vi "Load Reference.vi"(8 "error in (no error)":errorcluster, 10 "Reference":refnum<vi>, 11 "LargeScrollbar in":refnum<class "LargeScrollbar.lvclass">) -> (0 "error out":errorcluster, 3 "LargeScrollbar out":refnum<class "LargeScrollbar.lvclass">)   [LabVIEW 2015, in "LargeScrollbar.lvclass"]
doc: "The <b>Load Reference VI</b> is a dynamic dispatch VI that must be overwritten in every QControl Class and must <b>Call Parent Method</b>. This recursively loads the reference of the control to the data space for the Control Class up the inheritance hierarchy (class hierarchy). These references must be loaded in this way to use all of the built-in properties.\n\nThe reference input is the reference type needed for the control but is coerced to Generic. It should be cast back to the correct type before bundling into the class private data. The pre-casted \"Generic\" reference is wired as input to the <b>Call Parent Method</b>.\n<b> </b> <b> </b>\n©2016 Q Software Innovations, LLC (QSI)\nwritten by Quentin Alldredge\nproduced in LabVIEW 2015\n\nsupport@qsoftwareinnovations.com\nwww.qsoftwareinnovations.com\n\nAll rights reserved.\n\nRedistribution and use in source and binary forms, with or without modification, are permitted provided that the following conditions are met:\n\n * Redistributions of source code must retain the above copyright notice, this list of conditions and the following disclaimer.\n * Redistributions in binary form must reproduce the above copyright notice, this list of conditions and the following disclaimer in the documentation and/or other materials provided with the distribution.\n * Neither the name of Q Software Innovations, LLC. nor the names of its contributors may be used to endorse or promote products derived from this software without specific prior written permission.\n\nTHIS SOFTWARE IS PROVIDED BY THE COPYRIGHT HOLDERS AND CONTRIBUTORS \"AS IS\" AND ANY EXPRESS OR IMPLIED WARRANTIES, INCLUDING, BUT NOT LIMITED TO, THE IMPLIED WARRANTIES OF MERCHANTABILITY AND FITNESS FOR A PARTICULAR PURPOSE ARE DISCLAIMED. IN NO EVENT SHALL THE COPYRIGHT OWNER OR CONTRIBUTORS BE LIABLE FOR ANY DIRECT, INDIRECT, INCIDENTAL, SPECIAL, EXEMPLARY, OR CONSEQUENTIAL DAMAGES (INCLUDING, BUT NOT LIMITED TO, PROCUREMENT OF SUBSTITUTE GOODS OR SERVICES; LOSS OF USE, DATA, OR PROFITS; OR BUSINESS INTERRUPTION) HOWEVER CAUSED AND ON ANY THEORY OF LIABILITY, WHETHER IN CONTRACT, STRICT LIABILITY, OR TORT (INCLUDING NEGLIGENCE OR OTHERWISE) ARISING IN ANY WAY OUT OF THE USE OF THIS SOFTWARE, EVEN IF ADVISED OF THE POSSIBILITY OF SUCH DAMAGE."
uses:
  LargeScrollbar.lvclass
  LargeScrollbar.lvclass/LargeScrollbar.ctl
  Control/Control.lvclass
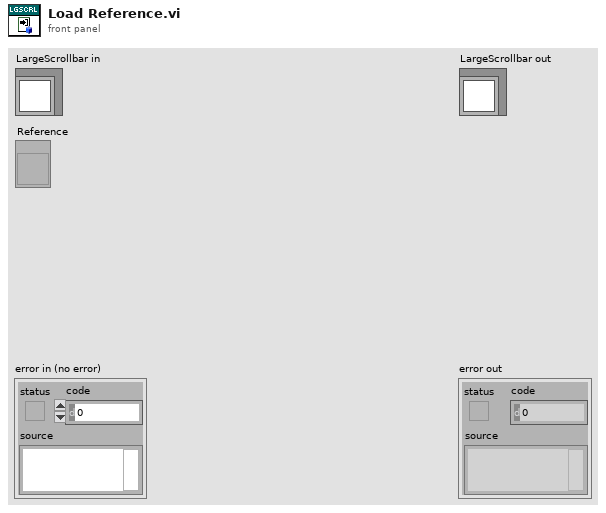
[diagram p1: front panel]
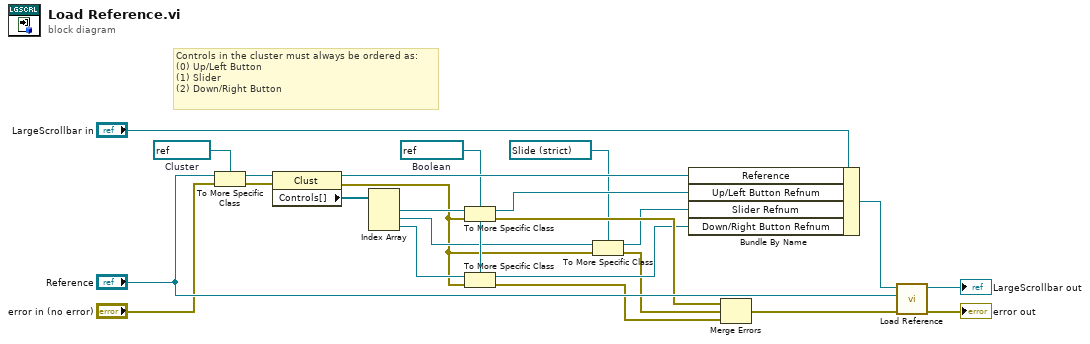
[diagram p0: block diagram]
diagram:
  w12 = refnum<vi> refnum  # Boolean
  w19 = refnum<vi> refnum  # Cluster
  # "Controls in the cluster must always be ordered as:\n(0) Up/Left Button\n(1) Slider\n(2) Down/Right Button"
  n1 = To More Specific Class(target class=w19, reference="Reference", error in="error in (no error)") -> (specific class reference=w18:refnum<vi>, error out=w15:errorcluster)
  n2 = property class="Clust"(reference=w18, error in=w15) -> (reference out=w16:refnum<vi>, error out=w9:errorcluster, "Controls[]"=w14:refnum<vi>[])
  n3 = Index Array(array=w14) -> (element #1=w13:refnum<vi>, element #2=w10:refnum<vi>, element #3=w11:refnum<vi>)  [unwired: 3 in]
  n4 = To More Specific Class(target class=w12, reference=w13, error in=w9) -> (specific class reference=w7:refnum<vi>, error out=w8:errorcluster)
  n5 = To More Specific Class(target class=w12, reference=w11, error in=w9) -> (specific class reference=w4:refnum<vi>, error out=w2:errorcluster)
  n6 = To More Specific Class(target class=refnum<vi> refnum ("Slide"), reference=w10, error in=w9) -> (specific class reference=w6:refnum<vi>, error out=w3:errorcluster)
  n7 = Bundle By Name(cluster="LargeScrollbar in", "Reference"=w16, "Up/Left Button Refnum"=w7, "Slider Refnum"=w6, "Down/Right Button Refnum"=w4) -> (w21:refnum<class "LargeScrollbar.lvclass">)
  n8 = Merge Errors(w8, w3, w2) -> (w1:errorcluster)
  n9 = call-parent "Load Reference.vi"("error in (no error)"=w1, "Reference"="Reference", "Control in"=w21) -> ("error out"=→"error out":errorcluster, "Control out"=→"LargeScrollbar out":refnum<class "LargeScrollbar.lvclass">)  [unwired: 7 in]
